vi "仿真2.vi"() -> ()   [LabVIEW 2018]
uses:
  <vilib>/Utility/file.llb/Write Delimited Spreadsheet (DBL).vi
panel:
  in  "?":enum32{"OFDM", "错误"}(tab)
  out "错误个数":dbl format="%#_13g"
  out "误比特率":dbl format="%#_13g"
  out "信噪比/dB":dbl format="%#_13g"
  out "已循环次数":i32
  in  "error in (no error)":errorcluster caption="错误输入"
  out "error out":errorcluster caption="错误输出"
  out "均衡后的星座图":cdb[](graph)
  out "理论4QAM星座图":cdb[](graph)
  out "输入比特流":i8[](array[numeric])
  in  "?":enum32{"幅值", "相位", "FFT{x}", "角度"}(tab)
  out "Magnitude":dbl[](graph)
  out "Phase":dbl[](graph)
  out "FFT{x}":dbl[](graph)
  out "角度":dbl[](graph)
  in  "?":enum32{"硬件参数", "调制参数"}(tab)
  in  "硬件参数":T1={"USRP IP Address"="NI2901", "IQ rate"=2000000.0, "carrier frequency"=450000000.0, "gain"=20.0, "active antenna"="RX2", "channel list"="0"} {"gain" format="%#_6f"; "carrier frequency" format="%#_6p"; "IQ rate" format="%#_6p"}
  in  "?":T2={"过采样因子"=20.0, "脉冲成形参数"={"调制类型"=enum."PSK", "脉冲成形滤波器"=enum."Raised Cosine", "滤波器参数"=0.5, "滤波长度 (码元)"=8.0}, "载波数"=128, "总比特数"=25600, "循环次数"=1000, "信噪比门限/dB"=15, "M-QAM (16)"=4} {"脉冲成形参数"."滤波器参数" format="%.2f"}
  out "输出比特流":i8[](array[numeric])
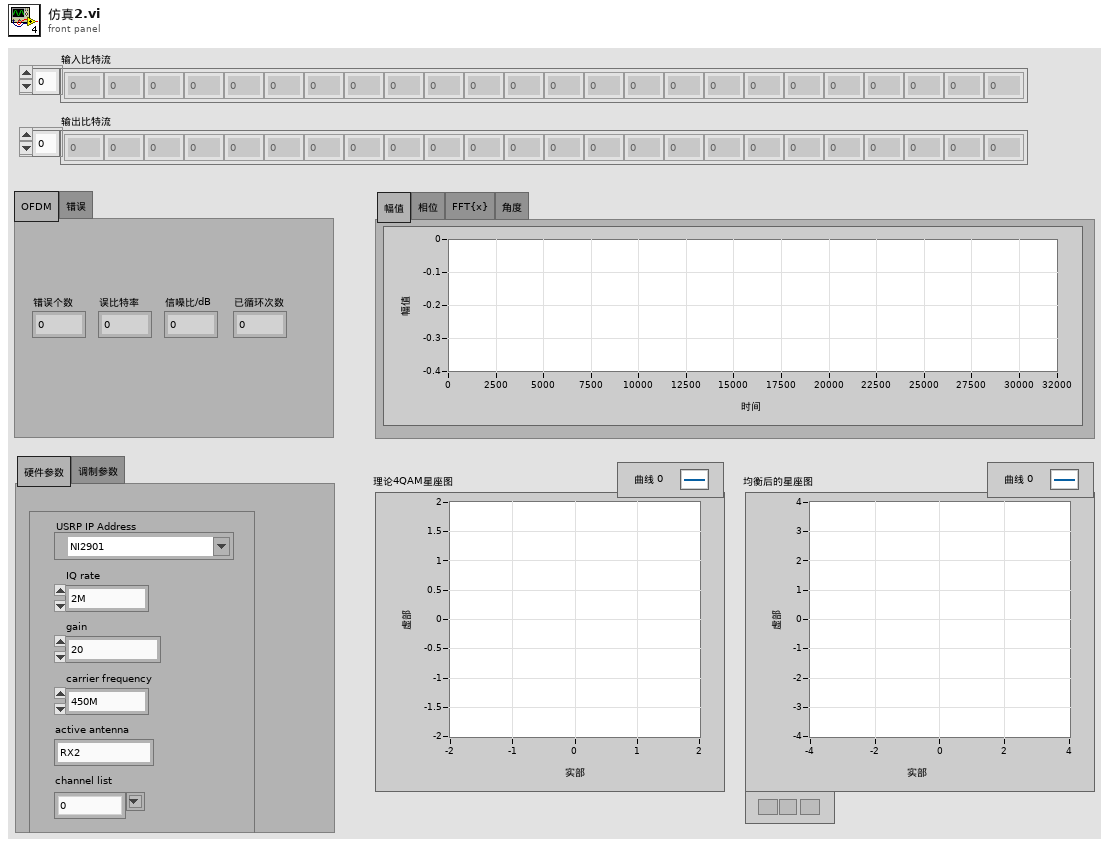
[diagram p1: front panel]
types:
  T1 = cluster{"USRP IP Address":refnum<k15>, "IQ rate":dbl, "carrier frequency":dbl, "gain":dbl, "active antenna":string, "channel list":string}
  T2 = cluster{"过采样因子":dbl, "脉冲成形参数":cluster{"调制类型":enum16{"FSK", "PSK", "QAM", "MSK", "PAM", "ASK", "CPM"}, "脉冲成形滤波器":enum16{"none", "Raised Cosine", "Root Raised Cos", "Gaussian"}, "滤波器参数":dbl, "滤波长度 (码元)":dbl}, "载波数":i32, "总比特数":i32, "循环次数":i32, "信噪比门限/dB":i32, "M-QAM (16)":i32}
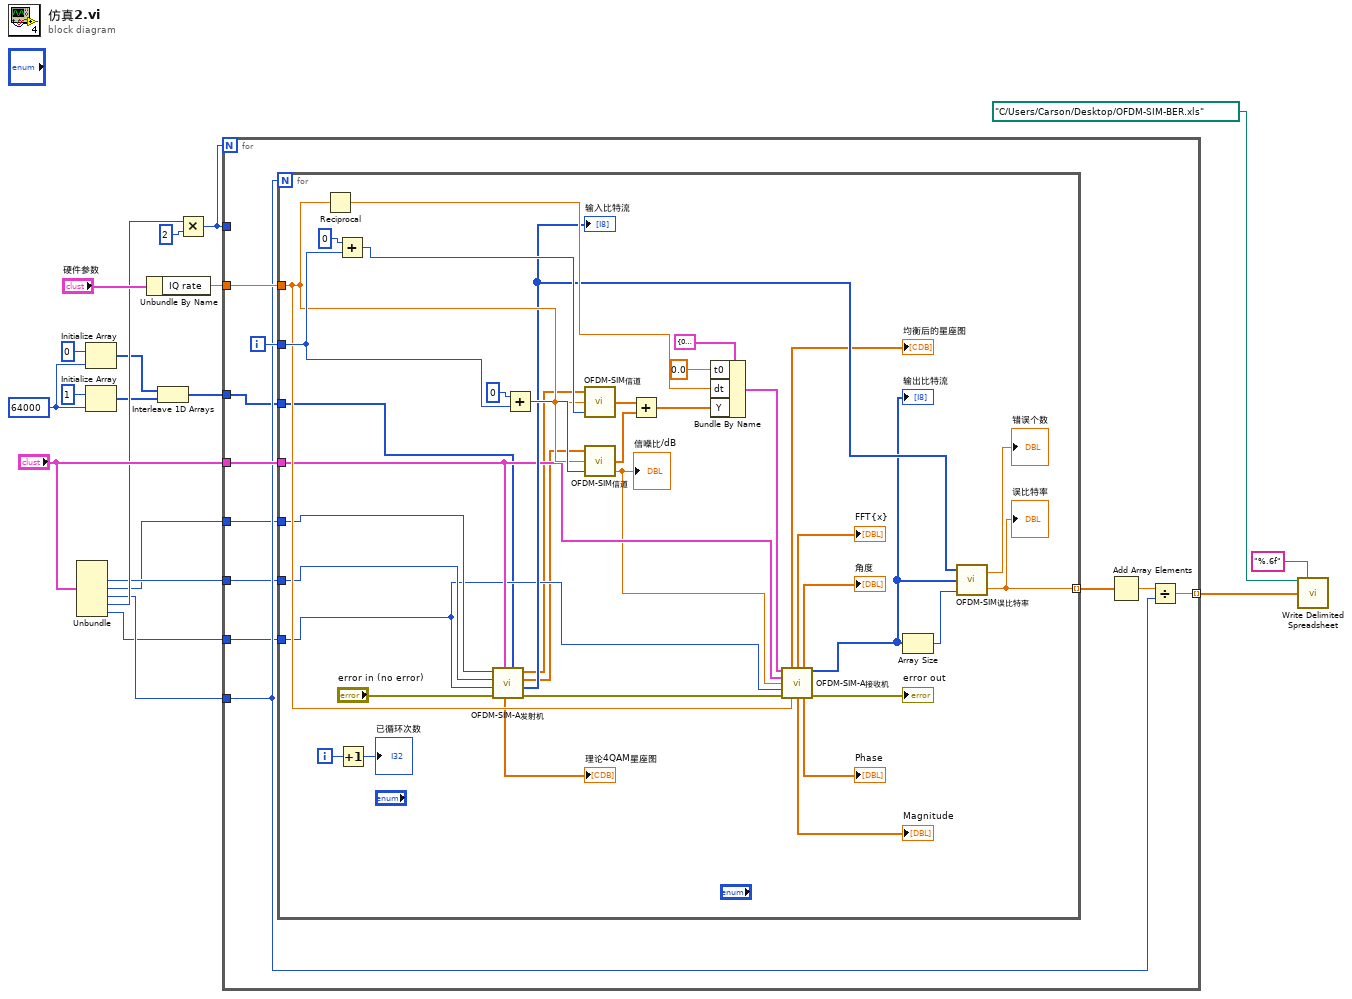
[diagram p0: block diagram]
diagram:
  w5 = 64000
  n1 = Unbundle("?") -> ("载波数"=w10:i32, "总比特数"=w9:i32, "循环次数"=w11:i32, "信噪比门限/dB"=w12:i32, "M-QAM (16)"=w8:i32)  [unwired: 2 out]
  n2 = Initialize Array(0, w5) -> (w3:i32[])
  n3 = Initialize Array(1, w5) -> (w4:i32[])
  n4 = Unbundle By Name("硬件参数") -> ("IQ rate"=w16:dbl)
  n5 = Interleave 1D Arrays(w3, w4) -> (w2:i32[])
  n6 = Multiply(x=w12, y=2) -> (x*y=w14:i32)
  n7 = for {
    N: w14 -> [_]
    tunnel: [w27] -> w19 mode=indexing
    tunnel: w16 -> [w30]
    tunnel: w14 -> [_]
    tunnel: "?" -> [w25]
    tunnel: w11 -> [w24]
    tunnel: w10 -> [w23]
    tunnel: w9 -> [w22]
    tunnel: w8 -> [w21]
    tunnel: w2 -> [w20]
    i -> [w29]
    n8 = for {
      N: w24 -> [_]
      tunnel: [w51] -> w28 mode=indexing
      tunnel: w30 -> [w54]
      tunnel: w29 -> [w57]
      tunnel: w25 -> [w43]
      tunnel: w23 -> [w45]
      tunnel: w22 -> [w44]
      tunnel: w21 -> [w42]
      tunnel: w20 -> [w39]
      i -> [w36]
      n9 = Reciprocal(x=w54) -> (1/x=w61:dbl)
      n10 = Add(x=0, y=w57) -> (x+y=w63:i32)
      n11 = Increment(x=w36) -> (x+1=→"已循环次数":i32)
      n12 = call "OFDM-SIM-A发射机.vi"("SIM比特"=w39, 6:w43, "error in (no error)"="error in (no error)", "M-QAM (16)"=w42, "载波数"=w45, "总比特数"=w44) -> ("error out"=w55:errorcluster, "输入比特流"=w52:i8[], "天线2发射信号"=w34:cdb[], "天线1发射信号"=w33:cdb[], "理论4QAM星座图"=→"理论4QAM星座图":cdb[])
      "输入比特流" <- w52
      n13 = Add(x=0, y=w57) -> (x+y=w65:i32)
      n14 = call "OFDM-SIM信道.vi"("数值"=w63, "采样率"=w54, "发射信号"=w33) -> ("接收信号2"=w32:cdb[])  [unwired: 2 out]
      n15 = call "OFDM-SIM信道.vi"("数值"=w65, "采样率"=w54, "发射信号"=w34) -> ("信噪比"=w41:dbl, "接收信号2"=w31:cdb[])  [unwired: 1 out]
      "信噪比/dB" <- w41
      n16 = Add(x=w32, y=w31) -> (x+y=w59:cdb[])
      n17 = Bundle By Name(cluster=cluster{"t0":dbl, "dt":dbl, "Y":cdb[]} {"t0"=0.0, "dt"=1.0, "Y"=[]} ("IQ data (complex) in"), "t0"=0.0, "dt"=w61, "Y"=w59) -> (w56:cluster{"t0":dbl, "dt":dbl, "Y":cdb[]})
      n18 = call "OFDM-SIM-A接收机.vi"("input complex waveform"=w56, 5:w43, "信噪比"=w41, "M-QAM"=w42, "error in (no error)"=w55, "IQ采样率"=w54) -> ("均衡后的星座图"=→"均衡后的星座图":cdb[], "FFT{x}"=→"FFT{x}":dbl[], "角度"=→"角度":dbl[], "输出比特流"=w38:i8[], "Magnitude"=→"Magnitude":dbl[], "Phase"=→"Phase":dbl[], "error out"=→"error out":errorcluster)  [unwired: 3 in]
      "输出比特流" <- w38
      n19 = Array Size(array=w38) -> (size(s)=w37:i32)
      n20 = call "OFDM-SIM误比特率.vi"("比特数"=w37, "输出比特"=w38, "输入比特"=w52) -> ("误比特率"=w51:dbl, "错误个数"=→"错误个数":dbl)
      "误比特率" <- w51
    }
    n21 = Add Array Elements(numeric array=w28) -> (sum=w26:dbl)
    n22 = Divide(x=w26, y=w24) -> (x/y=w27:dbl)
  }
  n23 = call-poly <vilib>:"Write Delimited Spreadsheet.vi"("file path (dialog if empty)"=path "C:/Users/Carson/Desktop/OFDM-SIM-BER.xls", "format (%.3f)"="%.6f", "1D data"=w19) -> ()  [unwired: 11 in, 2 out]
